vi "List_Processes.vi"(7 "Process filter":string="Lab", 8 "error in (no error)":errorcluster) -> (0 "error out":errorcluster, 4 "Match?":bool=TRUE, 5 "Open Proceesses":string[](array[string])=["C:\\Program Files\\National Instruments\\LabVIEW 8.2\\LabVIEW.exe"])   [LabVIEW 2018]
uses:
  psapi.dll
  KERNEL32.DLL
panel:
  out "process handle":u32=23160
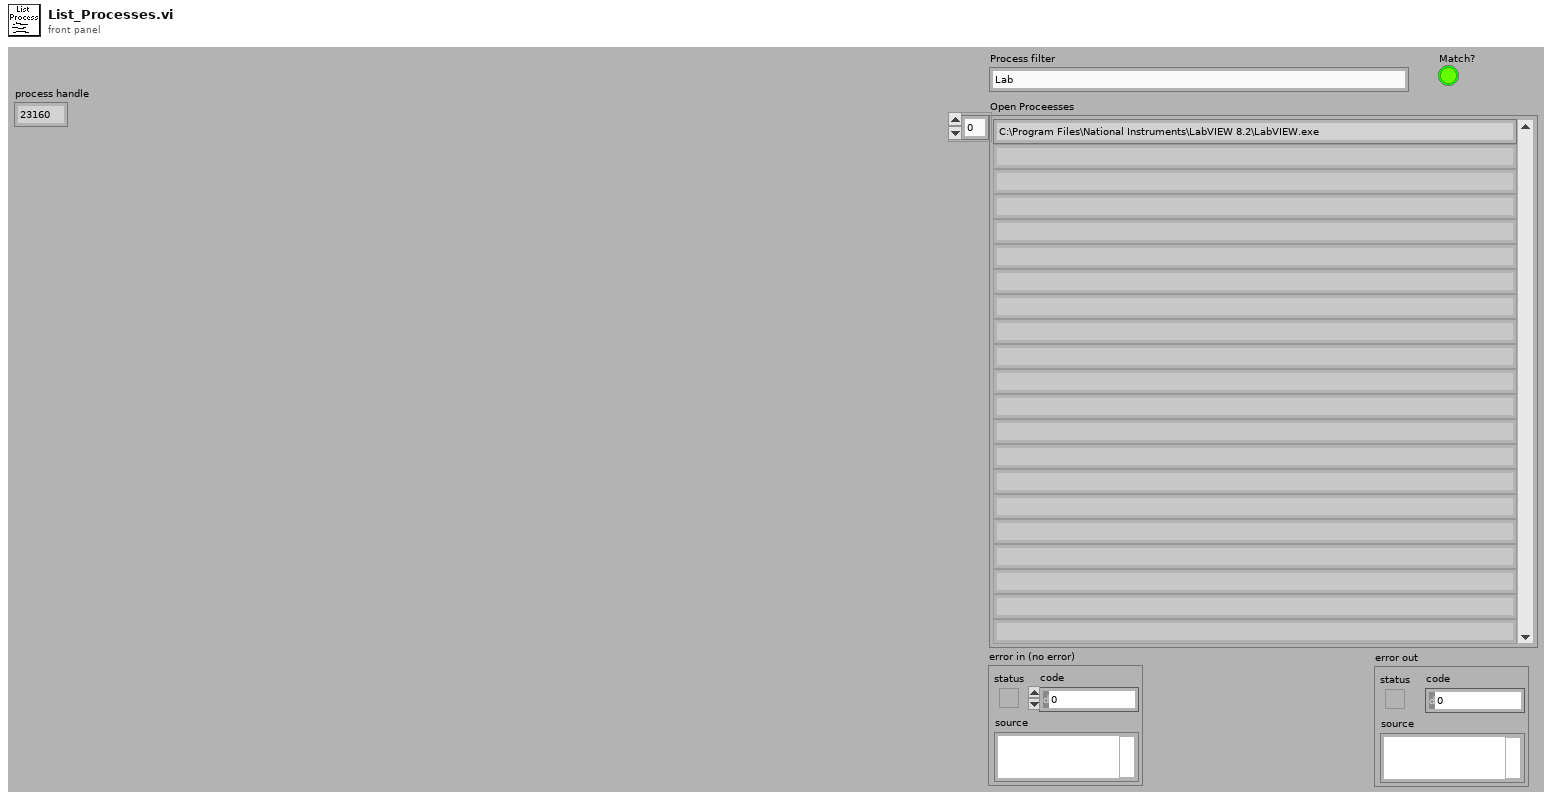
[diagram p1: front panel]
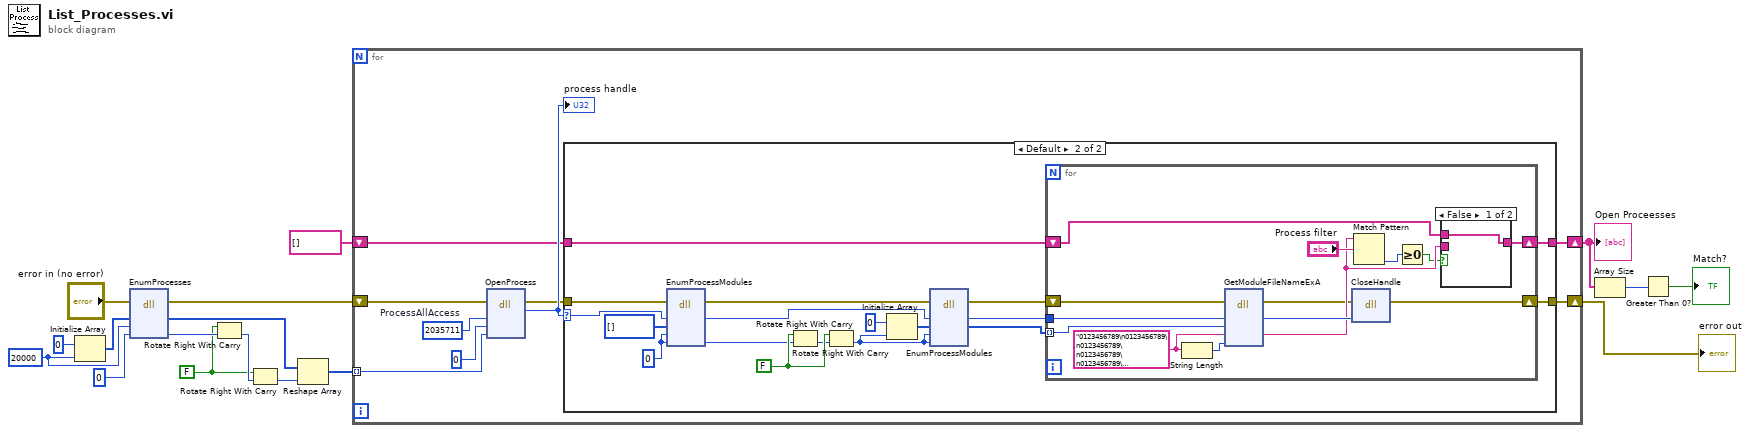
[diagram p0: block diagram]
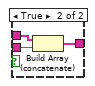
[diagram p3: hidden frame]
diagram:
  w8 = FALSE ("carry")
  w15 = 20000
  n1 = Initialize Array(u32 0, w15) -> (w16:u32[])
  n2 = dll-call lib="psapi.dll" fn="EnumProcesses"(error in="error in (no error)", "lpidProcess"=w16, "cb"=w15, "cbNeeded"=u32 0) -> (error out=w2:errorcluster, "lpidProcess"=w12:u32[], "cbNeeded"=w13:u32)  [unwired: 3 in, 2 out]
  n3 = Rotate Right With Carry(2:w13, 3:w8) -> (0:w10:u32)  [unwired: 1 out]
  n4 = Rotate Right With Carry(2:w10, 3:w8) -> (0:w9:u32)  [unwired: 1 out]
  n5 = Reshape Array(w12, w9) -> (w11:u32[])
  n6 = for {
    tunnel: w11 -> [w25] mode=indexing
    shift-right: [w21] -> w6
    shift-left: string[] [] -> [w22]
    shift-right: [w18] -> w1
    shift-left: w2 -> [w20]
    w23 = 2035711  # ProcessAllAccess
    n7 = dll-call lib="kernel32.dll" fn="OpenProcess"(error in=w20, "dwDesiredAccessas"=w23, "bInheritHandle"=0, "dwProcId"=w25) -> (error out=w19:errorcluster, w24:u32)  [unwired: 5 in, 1 out]
    "process handle" <- w24
    n8 = case shown="Default" w24 {
      selector: w24 -> [_ w46]
      tunnel: [w28 w34] -> w21
      tunnel: w22 -> [w28 w33]
      tunnel: w19 -> [w27 w32]
      tunnel: [w27 w29] -> w18
      frame 0 {
      }
      frame Default {
        w42 = FALSE ("carry")
        w45 = 0 ("cbNeeded")
        n9 = dll-call lib="psapi.dll" fn="EnumProcessModules"(error in=w32, "hProcesses"=w46, "lphModule"=u32[] [], "cb"=w45, "cbNeeded"=w45) -> (error out=w31:errorcluster, "hProcesses"=w37:u32, "cbNeeded"=w40:i32)  [unwired: 4 in, 2 out]
        n10 = Rotate Right With Carry(2:w40, 3:w42) -> (0:w41:i32)  [unwired: 1 out]
        n11 = Rotate Right With Carry(2:w41, 3:w42) -> (0:w38:i32)  [unwired: 1 out]
        n12 = Initialize Array(u32 0, w38) -> (w39:u32[])
        n13 = dll-call lib="psapi.dll" fn="EnumProcessModules"(error in=w31, "hProcesses"=w37, "lphModule"=w39, "cb"=w38, "cbNeeded"=w38) -> (error out=w30:errorcluster, "hProcesses"=w36:u32, "lphModule"=w35:u32[])  [unwired: 3 in, 3 out]
        n14 = for {
          tunnel: w36 -> [w58]
          tunnel: w35 -> [w57] mode=indexing
          shift-right: [w54] -> w34
          shift-left: w33 -> [w55]
          shift-right: [w47] -> w29
          shift-left: w30 -> [w49]
          w59 = "0123456789\n0123456789\n0123456789\n0123456789\n0123456789\n01234567890123456789\n0123456789\n0123456789\n0123456789\n0123456789\n01234567890123456789\n0123456789\n0123456789\n0123456789\n0123456789\n01234567890123456789\n0123456789\n0123456789\n0123456789\n0123456789\n01234567890123456789\n0123456789\n0123456789\n0123456789\n0123456789\n01234567890123456789\n0123456789\n0123456789\n0123456789\n0123456789\n0123456789"
          n15 = String Length(string=w59) -> (length=w60:i32)
          n16 = dll-call lib="psapi.dll" fn="GetModuleFileNameExA"(error in=w49, "hProcess"=w58, "hModule"=w57, "ModuleName"=w59, "nSize"=w60) -> (error out=w48:errorcluster, "hProcess"=w56:u32, "ModuleName"=w52:string)  [unwired: 4 in, 2 out]
          n17 = dll-call lib="kernel32.dll" fn="CloseHandle"(error in=w48, "Handle"=w56) -> (error out=w47:errorcluster)  [unwired: 3 in, 2 out]
          n18 = Match Pattern(string=w52, regular expression="Process filter") -> (offset past match=w51:i32)  [unwired: 4 out]
          n19 = Greater Or Equal To 0?(x=w51) -> (x >= 0?=w50:bool)
          n20 = case shown="False" w50 {
            tunnel: w55 -> [w61 w64]
            tunnel: [w61 w63] -> w54
            tunnel: w52 -> [_ w62]
            frame False {
            }
            frame True {
              n21 = Build Array (concatenate)(w64, w62) -> (w63:string[])
            }
          }
        }
      }
    }
  }
  "Open Proceesses" <- w6
  "error out" <- w1
  n22 = Array Size(array=w6) -> (size(s)=w5:i32)
  n23 = Greater Than 0?(x=w5) -> (x > 0?=→"Match?":bool)
